vi "grain bin indicator debug 2.vi"() -> ()   [LabVIEW 2020]
uses:
  Type Defs/Bin Indicator Type Def.ctl
panel:
  in  "Tab Control 3":enum32{"Page 1"}(tab)
  in  "Button 10":bool
  in  "Button 9":bool
  in  "Button 8":bool
  in  "Button 7":bool
  out "Fault":bool=TRUE
  out "Running":bool=TRUE
  in  "Button 6":bool
  out "Dryer_Numeric 2":u16=140 caption="bu"
  in  "Tab Control":enum32{"Page 1"}(tab)
  out "Overload":bool=TRUE
  out "Running":bool=TRUE
  in  "Button 5":bool
  in  "Tab Control 2":enum32{"Page 1"}(tab)
  out "WB_Numeric":u16=400 caption="bu"
  out "WS_Numeric":u16=246 caption="bu"
  out "Dryer_Numeric":u16=140 caption="bu"
  out "DB_Numeric":u16=330 caption="bu"
  out "DB_Scale":bool
  out "DB_Background":bool=TRUE
  in  "Dry Bin Level":u16=330
  out "DB_Fan":bool=TRUE
  out "DB_Drag":bool=TRUE
  out "Fan 2":bool=TRUE
  out "Drag 2":bool=TRUE
  out "Fan 3":bool
  out "Fan 4":bool=TRUE
  out "Drag 3":bool
  out "Drag 4":bool=TRUE
  out "Leg":bool
  out "DB Top Feed":bool
  in  "Dryer Level":u16=140
  in  "Wet Bin Level":u16=400
  in  "Wet Silo Level":u16=246
  out "Dryer_Scale":bool
  out "Dryer_Background":bool=TRUE
  out "WB_Scale":bool
  out "WB_Background":bool=TRUE
  out "WS_Scale":bool
  out "WS_Background":bool=TRUE
  in  "Button":bool
  in  "Button 2":bool
  in  "Button 3":bool
  in  "Button 4":bool
  # "rpm"
  # "DRY BIN"
  # "WET SILO"
  # "CONTROL\nROOM"
  # "DRY BIN\nTOP FEED"
  # "LEG"
  # "DRYER /\nDRYER BIN"
  # "WET BIN"
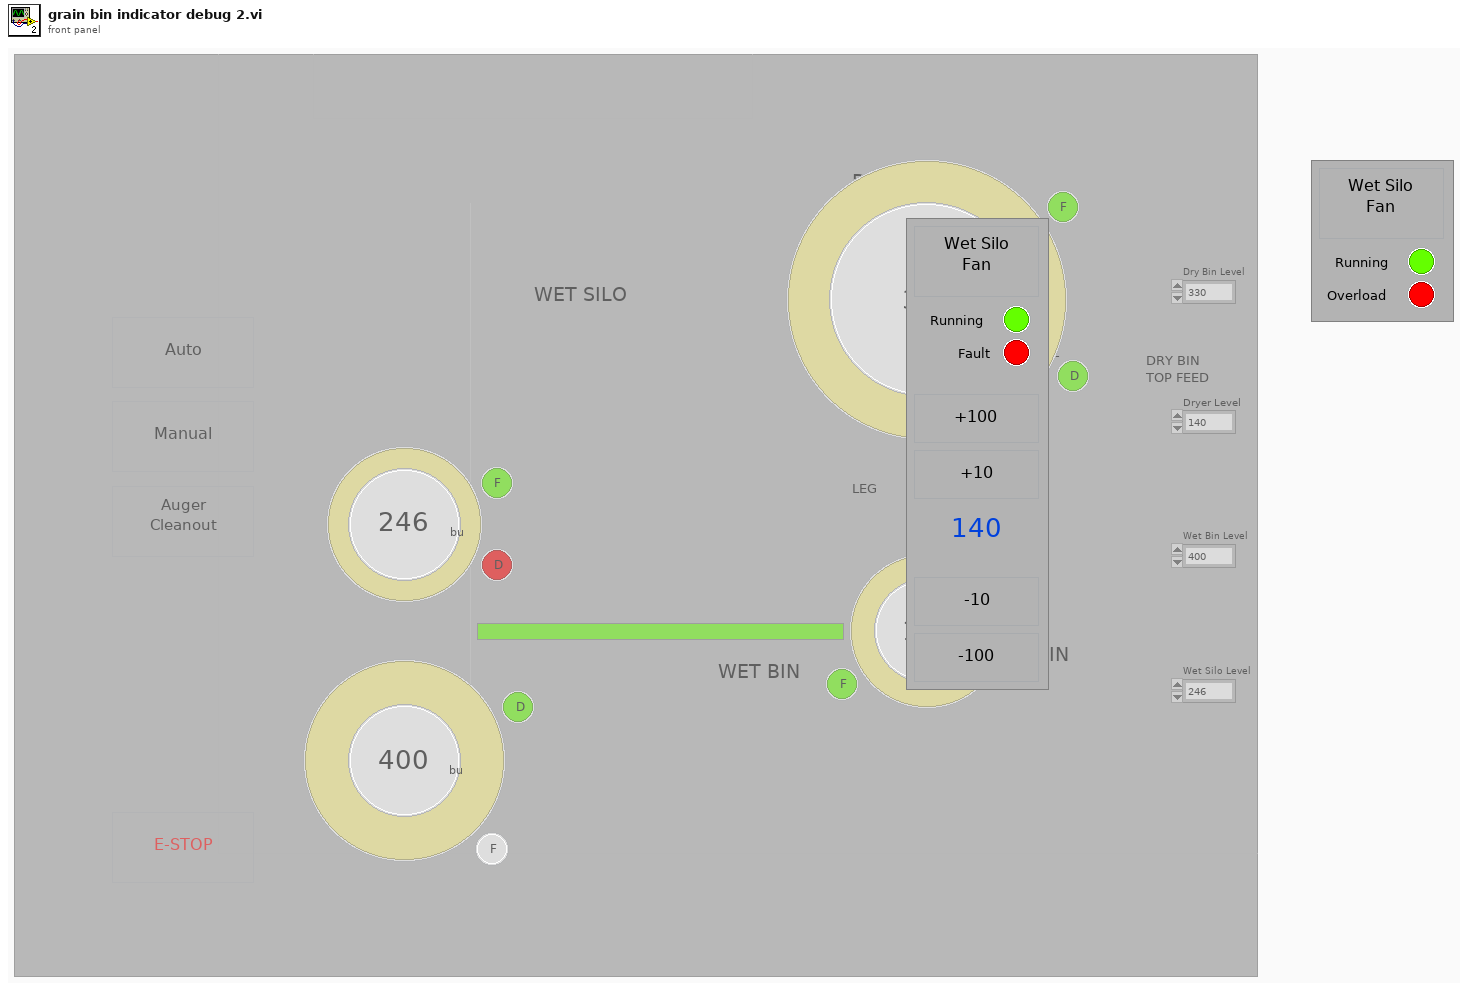
[diagram p1: front panel]
types:
  T1 = typedef "Bin Indicator Type Def.ctl" = cluster{"Scale":refnum<vi>, "Background":refnum<vi>, "Numeric":refnum<vi>, "Bin Max":u16}
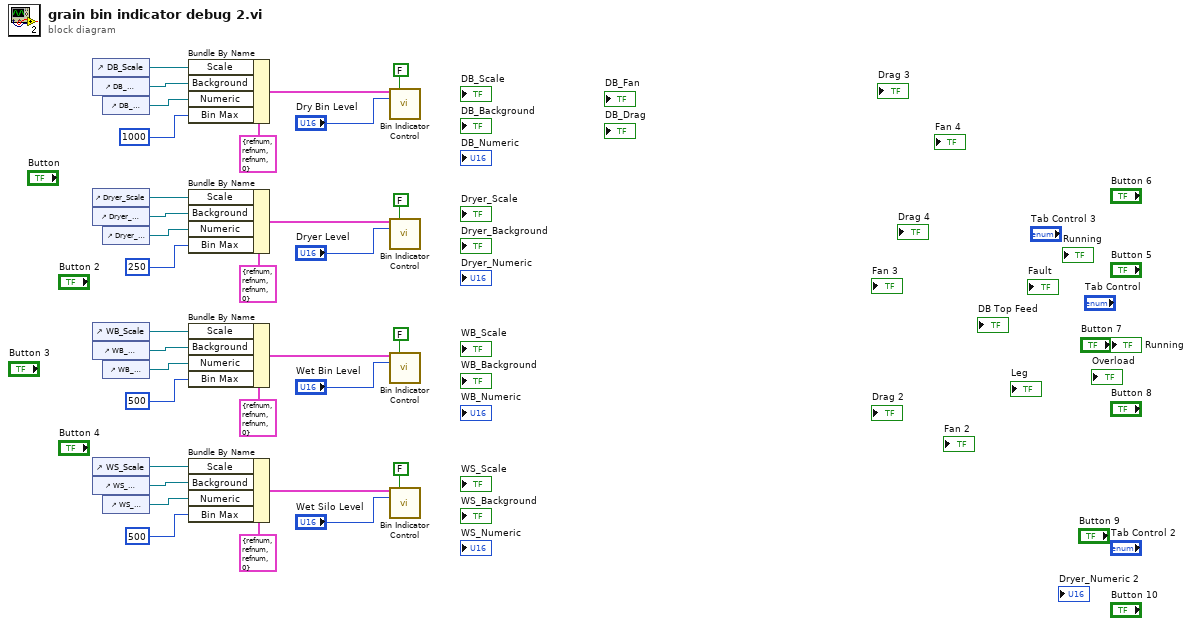
[diagram p0: block diagram]
diagram:
  n1 = control-ref of="DB_Scale"() -> (w31:refnum<vi>)
  n2 = control-ref of="DB_Background"() -> (w30:refnum<vi>)
  n3 = control-ref of="Dryer_Scale"() -> (w18:refnum<vi>)
  n4 = control-ref of="Dryer_Background"() -> (w19:refnum<vi>)
  n5 = control-ref of="WB_Scale"() -> (w15:refnum<vi>)
  n6 = control-ref of="WB_Background"() -> (w14:refnum<vi>)
  n7 = control-ref of="WS_Scale"() -> (w2:refnum<vi>)
  n8 = control-ref of="WS_Background"() -> (w3:refnum<vi>)
  n9 = control-ref of="DB_Numeric"() -> (w29:refnum<vi>)
  n10 = control-ref of="Dryer_Numeric"() -> (w20:refnum<vi>)
  n11 = control-ref of="WB_Numeric"() -> (w13:refnum<vi>)
  n12 = control-ref of="WS_Numeric"() -> (w4:refnum<vi>)
  n13 = Bundle By Name(cluster=T1 {"Scale"=refnum, "Background"=refnum, "Numeric"=refnum, "Bin Max"=0} ("Bin Indicator Refs"), "Scale"=w31, "Background"=w30, "Numeric"=w29, "Bin Max"=u16 1000) -> (w28:T1)
  n14 = Bundle By Name(cluster=T1 {"Scale"=refnum, "Background"=refnum, "Numeric"=refnum, "Bin Max"=0} ("Bin Indicator Refs"), "Scale"=w18, "Background"=w19, "Numeric"=w20, "Bin Max"=u16 250) -> (w21:T1)
  n15 = Bundle By Name(cluster=T1 {"Scale"=refnum, "Background"=refnum, "Numeric"=refnum, "Bin Max"=0} ("Bin Indicator Refs"), "Scale"=w15, "Background"=w14, "Numeric"=w13, "Bin Max"=u16 500) -> (w12:T1)
  n16 = Bundle By Name(cluster=T1 {"Scale"=refnum, "Background"=refnum, "Numeric"=refnum, "Bin Max"=0} ("Bin Indicator Refs"), "Scale"=w2, "Background"=w3, "Numeric"=w4, "Bin Max"=u16 500) -> (w5:T1)
  n17 = call "Bin Indicator Control.vi"("Bin Indicator Refs"=w28, "Init (F)"=FALSE, "Bin Level"="Dry Bin Level") -> ()  [unwired: 13 in]
  n18 = call "Bin Indicator Control.vi"("Bin Indicator Refs"=w21, "Init (F)"=FALSE, "Bin Level"="Dryer Level") -> ()  [unwired: 13 in]
  n19 = call "Bin Indicator Control.vi"("Bin Indicator Refs"=w12, "Init (F)"=FALSE, "Bin Level"="Wet Bin Level") -> ()  [unwired: 13 in]
  n20 = call "Bin Indicator Control.vi"("Bin Indicator Refs"=w5, "Init (F)"=FALSE, "Bin Level"="Wet Silo Level") -> ()  [unwired: 13 in]
